vi "Freq2Mel.vi"(11 "F":dbl) -> (3 "Mel":dbl)   [LabVIEW 2020]
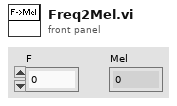
[diagram p1: front panel]
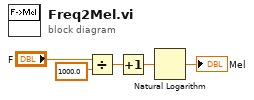
[diagram p0: block diagram]
diagram:
  n1 = Divide(x="F", y=1000.0) -> (x/y=w3:dbl)
  n2 = Increment(x=w3) -> (x+1=w4:dbl)
  n3 = Natural Logarithm(1:w4) -> (0:→"Mel":dbl)
